vi "Y Coil Magnetic field to Voltage (SubVI).vi"(11 "Magnetic field [µT]":dbl) -> (3 "Voltage Y":string)   [LabVIEW 2018]
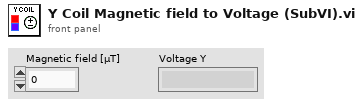
[diagram p1: front panel]
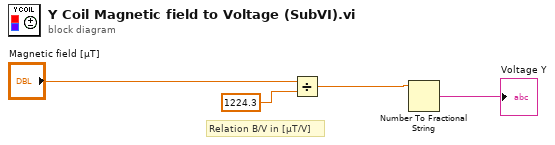
[diagram p0: block diagram]
diagram:
  # "Relation B/V in [µT/V]"
  n1 = Divide(x="Magnetic field [µT]", y=1224.3) -> (x/y=w3:dbl)
  n2 = Number To Fractional String(number=w3) -> (F-format string=→"Voltage Y":string)  [unwired: 3 in]
